vi "Convert BMP (1D to 2D).vi"(8 "error in (no error)":errorcluster, 10 "Matric Resolution In":i32=85, 11 "BMP Image Path":path) -> (0 "Colour Depth":i32, 1 "Resolution (Horizontal)":i32, 2 "2D Pixel Map":i32[][](array[numeric]), 3 "Total of Image Pixels":i32=89232, 4 "Pixels per LED":i32, 5 "Image Width (pixels)":i16, 6 "Resolution (Verticle)":i32, 7 "Image Height (pixels)":i16)   [LabVIEW 2014]
doc: "Load Bitmap file, and convert\nresulting 1D array of pixel\nintensities into a 2D pixel map"
panel:
  out "error out":errorcluster
  # "Image Information (Input)"
  # "Image Information (Output)"
  # "Dot Matrix Information (Output)"
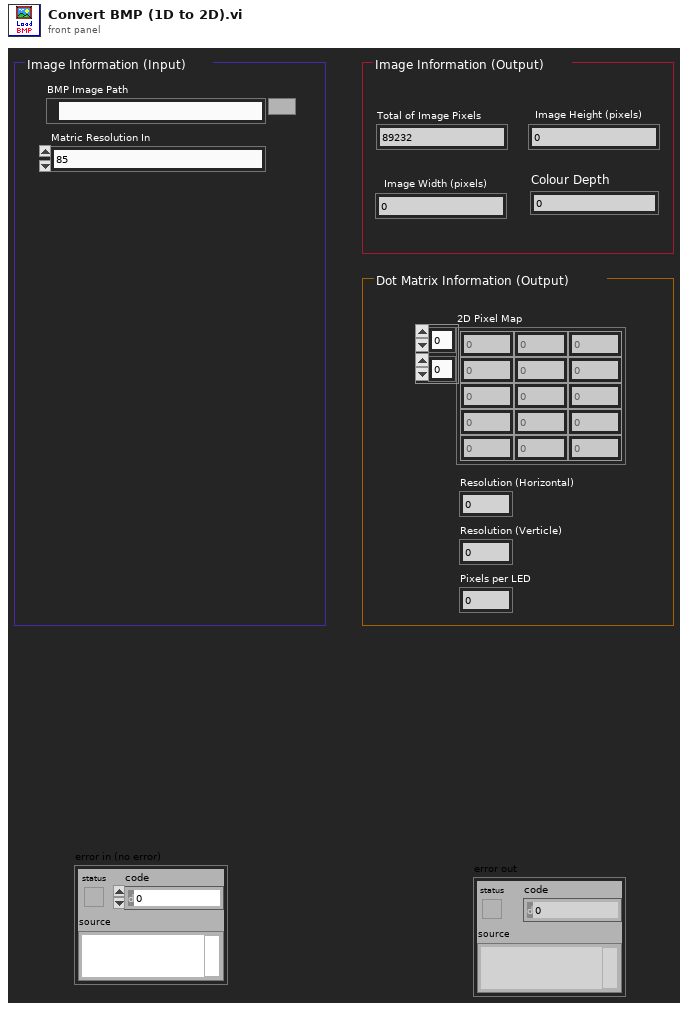
[diagram p1: front panel]
types:
  T1 = typedef "imagedata.ctl" = cluster{"image type":i32, "image depth":i32, "image":u8[], "mask":u8[], "colors":u32[], "Rectangle":cluster{"left":i16, "top":i16, "right":i16, "bottom":i16}}
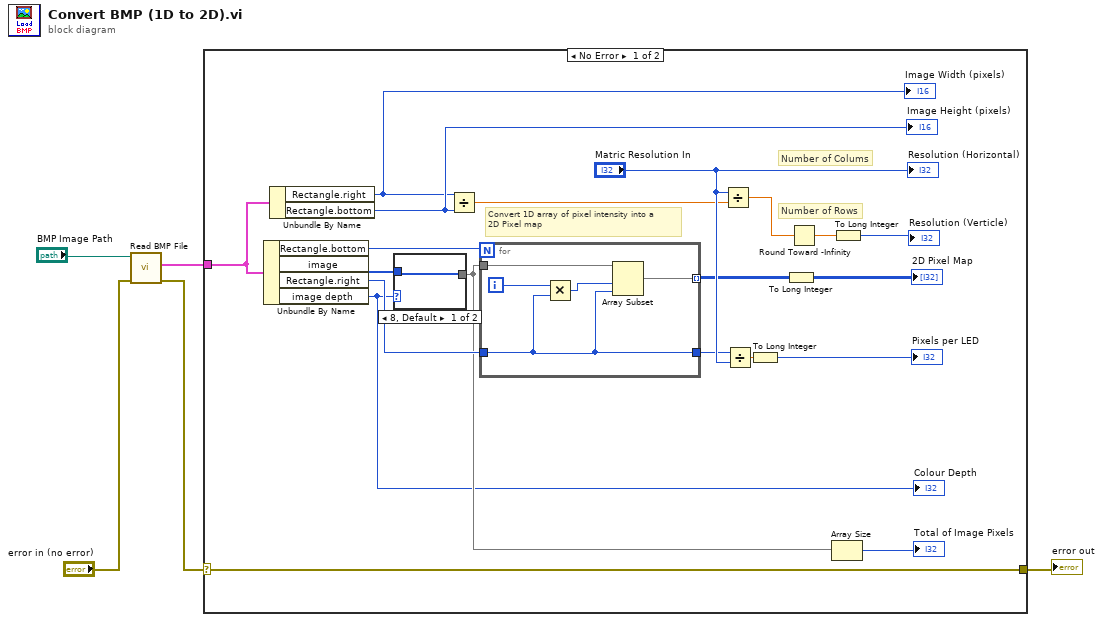
[diagram p0: block diagram]
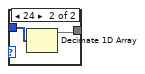
[diagram p2: hidden frame]
diagram:
  n1 = call <vilib>:"Read BMP File.vi"("error in (no error)"="error in (no error)", "path to BMP file"="BMP Image Path") -> ("error out"=w1:errorcluster, "image data"=w5:T1)  [unwired: 7 in, 1 out]
  n2 = case shown="No Error" w1 {
    selector: w1 -> [w9 w34]
    tunnel: w5 -> [w16 _]
    tunnel: [w9 w34] -> w2
    frame No Error {
      # "Convert 1D array of pixel intensity into a\n2D Pixel map"
      # "Number of Colums"
      # "Number of Rows"
      n3 = Unbundle By Name(w16) -> ("Rectangle.bottom"=w11:i16, "image"=w15:u8[], "Rectangle.right"=w10:i16, "image depth"=w6:i32)
      "Colour Depth" <- w6
      n4 = Unbundle By Name(w16) -> ("Rectangle.right"=w13:i16, "Rectangle.bottom"=w14:i16)
      "Image Width (pixels)" <- w13
      "Image Height (pixels)" <- w14
      n5 = case shown="8, Default" w6 {
        tunnel: w15 -> [w26 w28]
        tunnel: [w26 w27] -> w7
        frame 8, Default {
        }
        frame 24 {
          n6 = Decimate 1D Array(w28) -> (w27:u8[])  [unwired: 2 out]
        }
      }
      n7 = Divide(x=w13, y=w14) -> (x/y=w20:dbl)
      n8 = for {
        N: w11 -> [_]
        tunnel: w7 -> [w33]
        tunnel: w10 -> [w29]
        tunnel: [w30] -> w12 mode=indexing
        tunnel: [w29] -> w18
        i -> [w32]
        n9 = Multiply(x=w32, y=w29) -> (x*y=w31:i32)
        n10 = Array Subset(array=w33, index=w31, length=w29) -> (w30:u8[])
      }
      n11 = Divide(x="Matric Resolution In", y=w20) -> (x/y=w21:dbl)
      n12 = Divide(x=w18, y="Matric Resolution In") -> (x/y=w19:dbl)
      n13 = To Long Integer(number=w19) -> (32bit integer=→"Pixels per LED":i32)
      n14 = To Long Integer(number=w12) -> (32bit integer=→"2D Pixel Map":i32[][])
      n15 = Round Toward -Infinity(1:w21) -> (0:w23:dbl)
      n16 = Array Size(array=w7) -> (size(s)=→"Total of Image Pixels":i32)
      n17 = To Long Integer(number=w23) -> (32bit integer=→"Resolution (Verticle)":i32)
      "Resolution (Horizontal)" <- "Matric Resolution In"
    }
    frame Error {
    }
  }
  "error out" <- w2
